vi "Set Globals.vi"() -> (3 "Camera error out":errorcluster)   [LabVIEW 2018, in "Stresing_dual_cam.lvclass"]
uses:
  Stresing_dual_cam.lvclass
  board.vis/Globals.vi
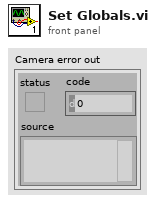
[diagram p1: front panel]
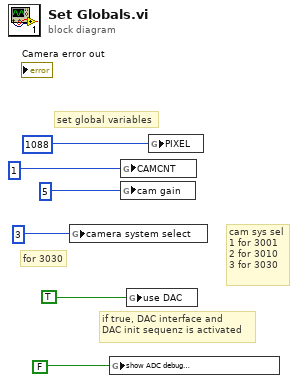
[diagram p0: block diagram]
diagram:
  # "if true, DAC interface and \nDAC init sequenz is activated"
  # "for 3030"
  # "set global variables"
  # "cam sys sel\n1 for 3001\n2 for 3010\n3 for 3030"
  n1 = global write "Globals.vi" "camera system select"(u8 3) -> ()
  n2 = global write "Globals.vi" "show ADC debug \ninterface"(FALSE) -> ()
  n3 = global write "Globals.vi" "CAMCNT"(u32 1) -> ()
  n4 = global write "Globals.vi" "cam gain"(u32 5) -> ()
  n5 = global write "Globals.vi" "use DAC"(TRUE) -> ()
  n6 = global write "Globals.vi" "PIXEL"(u32 1088) -> ()
